vi "To-simple-string.vi"(8 "error in (no error)":errorcluster, 11 "Move-Timer in":refnum<class "Move-Timer.lvclass">) -> (0 "error out":errorcluster, 2 "Action string":string, 3 "Move-Timer out":refnum<class "Move-Timer.lvclass">)   [LabVIEW 2013, in "PowderDeposition.lvlib" / "Move-Timer.lvclass"]
uses:
  Move-Timer.lvclass
  Move-Timer.lvclass/Move-Timer.ctl
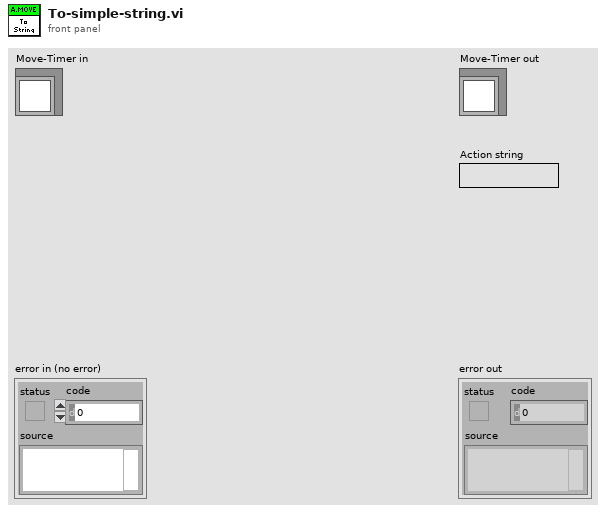
[diagram p1: front panel]
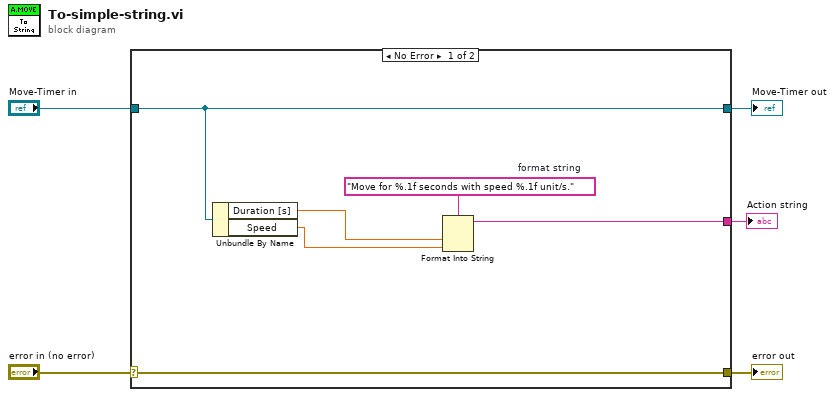
[diagram p0: block diagram]
diagram:
  n1 = case shown="No Error" "error in (no error)" {
    selector: "error in (no error)" -> [w11 w13]
    tunnel: [w11 w13] -> w4
    tunnel: [w10 w12] -> w2
    tunnel: "Move-Timer in" -> [w10 w12]
    tunnel: [w8 _] -> w1
    frame No Error {
      w9 = "Move for %.1f seconds with speed %.1f unit/s."  # format string
      n2 = Unbundle By Name(w10) -> ("Duration [s]"=w7:dbl, "Speed"=w6:dbl)
      n3 = Format Into String(format string=w9, w7, w6) -> (resulting string=w8:string)  [unwired: 2 in, 1 out]
    }
    frame Error {
    }
  }
  "error out" <- w4
  "Move-Timer out" <- w2
  "Action string" <- w1
